vi "Write to File.vi"(8 "error in (no error)":errorcluster, 10 "INI Ref":T1, 11 "Assertion Step in":refnum<class "Assertion Step.lvclass">) -> (0 "error out":errorcluster, 2 "INI Ref out":T1, 3 "Assertion Step out":refnum<class "Assertion Step.lvclass">)   [LabVIEW 2020, in "MacroAssert.lvlib" / "Assertion Step.lvclass"]
doc: "Writes associated parameters to the file identified by <B>INI Ref</B>."
uses:
  Assertion Step.lvclass
  C:/Users/User/Documents/LabVIEW Data/Projects/MacroAssert/source/Classes/Step/Step.lvclass
  <vilib>/Utility/config.llb/Config Data RefNum.ctl
  <vilib>/Utility/config.llb/Write Key (String).vi
  <vilib>/Utility/config.llb/Write Key (Boolean).vi
  Step/Step.lvclass
  MacroAssert.lvlib
  <vilib>/Utility/config.llb/NI_LVConfig.lvlib
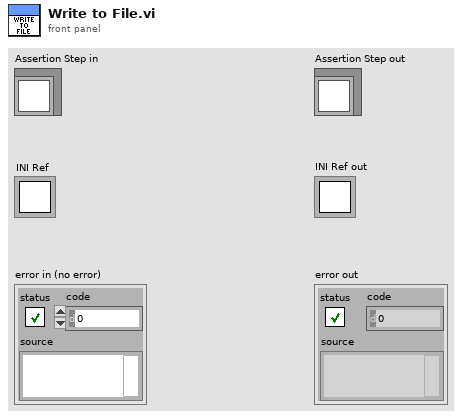
[diagram p1: front panel]
types:
  T1 = typedef "NI_LVConfig.lvlib/Config Data RefNum.ctl" = refnum<k1>
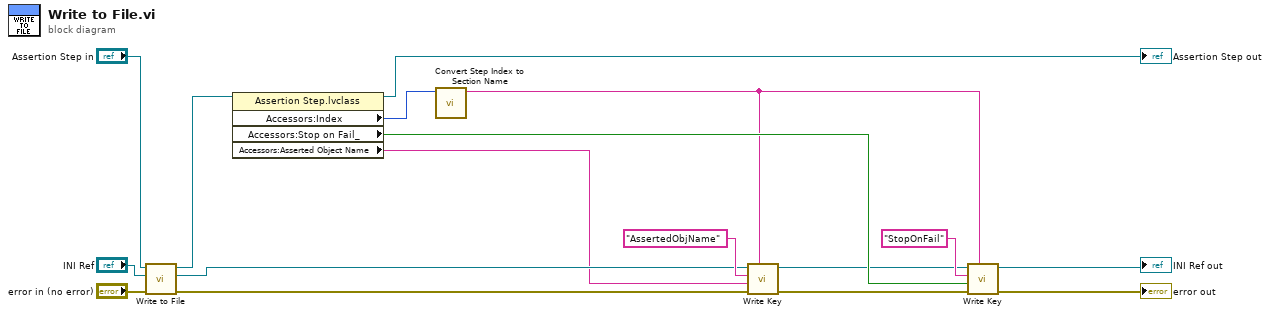
[diagram p0: block diagram]
diagram:
  n1 = call-parent "Write to File.vi"("error in (no error)"="error in (no error)", "INI Ref"="INI Ref", "Step in"="Assertion Step in") -> ("error out"=w6:errorcluster, "INI Ref out"=w3:T1, "Step out"=w10:refnum<class "Assertion Step.lvclass">)  [unwired: 6 in]
  n2 = property class="Assertion Step.lvclass"(reference=w10) -> (reference out=→"Assertion Step out":refnum<class "Assertion Step.lvclass">, "Accessors:Index"=w11:i32, "Accessors:Stop on Fail_"=w8:bool, "Accessors:Asserted Object Name"=w1:string)  [unwired: 1 in, 1 out]
  n3 = call "Convert Step Index to Section Name.vi"("Step Index"=w11) -> ("Section Name"=w2:string)  [unwired: 10 in]
  n4 = call-poly <vilib>:"Write Key.vi"("section"=w2, "error in (no error)"=w6, "value"=w1, "key"="AssertedObjName", "refnum"=w3) -> ("error out"=w5:errorcluster, "refnum out"=w4:T1)  [unwired: 4 in, 1 out]
  n5 = call-poly <vilib>:"Write Key.vi"("section"=w2, "error in (no error)"=w5, "value"=w8, "key"="StopOnFail", "refnum"=w4) -> ("error out"=→"error out":errorcluster, "refnum out"=→"INI Ref out":T1)  [unwired: 4 in, 1 out]
